vi "CSM - Destroy Global Log Queue.vi"(8 "Error In":errorcluster caption="error in (no error)", 11 "Global Log Queue":refnum<queue>) -> (0 "error out":errorcluster)   [LabVIEW 2017, in "Communicable State Machine.lvlib"]
doc: "Releases the global log queue refnum.\n\n\n> [!NOTE] <b>CSM Global Log Functionality</b>\n>\n> The CSM Global Log functionality is used to view global log change events, serving scenarios such as debugging and monitoring.\n> The following is the information that can be logged:\n> - Module state modifications\n> - Inter-module message communication, including data returns\n> - Message completion records of asynchronous and synchronous messages, `AsyncMsg Complete` and `SyncMsg Complete`, which carry the response\n> - Module status publishing\n> - Module creation and destruction\n> - Module state registration and unregistration\n> - Error information handled by modules\n> - User-defined events\n>\n> Debugging tools are primarily developed based on the Global Log API. You can develop debugging tools according to your own needs.\n\n\n> [!NOTE] <b>CSM Global Log Acquisition Methods</b>\n>\n> CSM provides two methods for acquiring global logs: Queue and Event. The Queue processing method is recommended because the queue interface is more efficient and offers greater flexibility in selecting log processing schemes based on the number of accumulated logs in the queue.\n\n\n<b>Reference Examples</b>:\n- `4. Advance Examples\\Filter From Source(Queue).vi`\n- `4. Advance Examples\\Filter From Subscriber(Queue).vi`\n\n-- <b>Controls</b> --\n- <b>Global Log Queue</b>: Global log queue refnum."
uses:
  Communicable State Machine.lvlib
  _Support/Typedef/_CSM_GlobalLog_MSG.ctl
  _Support/Typedef/_CSM_Response Source Message.ctl
  _Support/Typedef/_CSM_GlobalLog_MSG_TYPE.ctl
  _Support/ChangeFlag/ChangeFlag-Write.vi
  Utility/Random Change Flag.vi
  _Support/ChangeFlag/ChangeFlagDB.vi
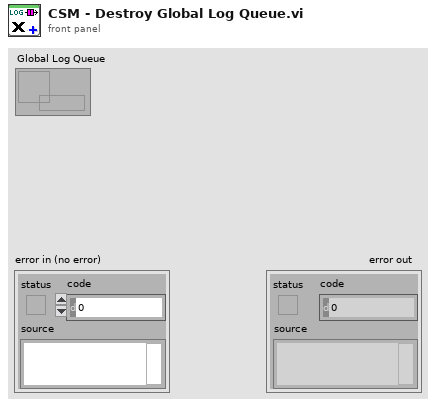
[diagram p1: front panel]
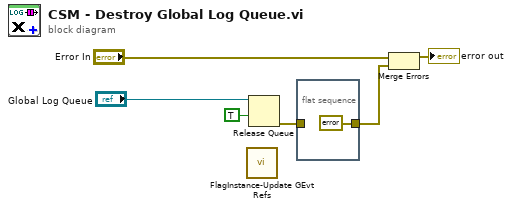
[diagram p0: block diagram]
diagram:
  n1 = call "FlagInstance-Update GEvt Refs.vi"() -> ()  [unwired: 10 in, 2 out]
  n2 = Release Queue(queue="Global Log Queue", force destroy? (F)=TRUE) -> (error out=w2:errorcluster)  [unwired: 1 in, 2 out]
  n3 = flat-sequence {
    tunnel: [errorcluster {"status"=FALSE, "code"=0, "source"=""} ("error out")] -> w4
    tunnel: w2 -> [_]
    frame #0 {
    }
  }
  n4 = Merge Errors("Error In", w4) -> (→"error out":errorcluster)
